vi "Param Sweep Dialog.vi"(8 "error in":errorcluster, 10 "Sweeps In":T1[](array[typedef])) -> (0 "error out":errorcluster, 1 "Cancelled?":bool, 2 "Sweeps out":T1[](array[typedef]), 4 "Movies to acquire":u32=1)   [LabVIEW 2023]
uses:
  Resources/Type Defs/Param Sweep.ctl
  896b73e1-52d9-41ed-b2a6-3a6588fcdd74.vi
panel:
  in  "Values":u32[](array[numeric])
  in  "Parameter":enum16{"Laser Power (mW)", "Exposure Time (ms)"}(ring)
  in  "Cancel":bool caption="Boolean 2"
  in  "Ok":bool caption="Boolean"
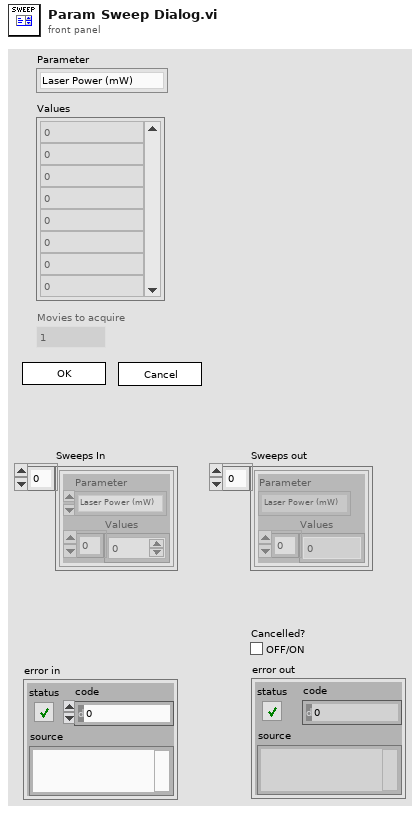
[diagram p1: front panel]
types:
  T1 = typedef "Param Sweep.ctl" = cluster{"Parameter":enum16{"Laser Power (mW)", "Exposure Time (ms)"}, "Values":u32[]}
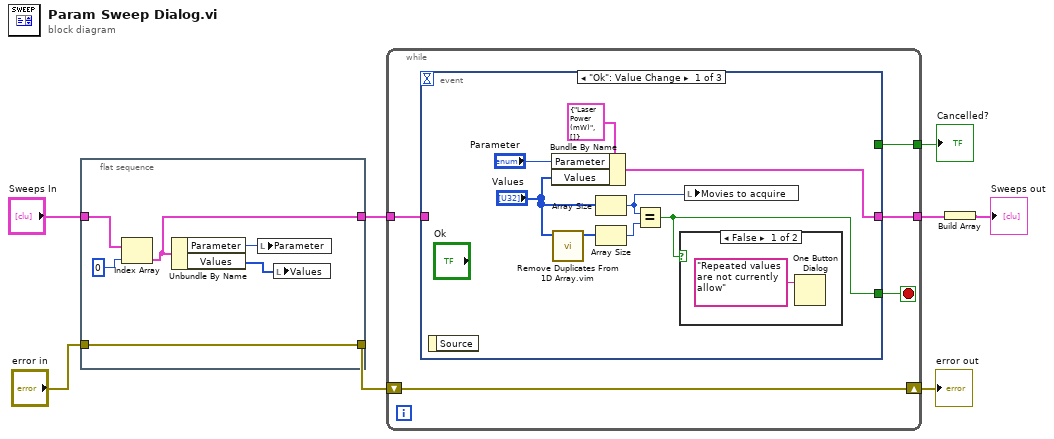
[diagram p0: block diagram]
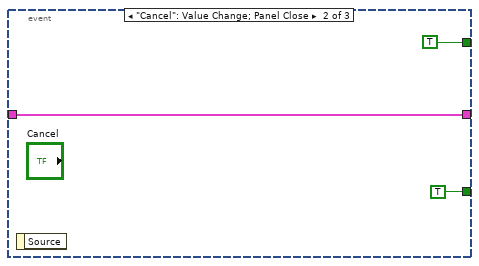
[diagram p3: hidden frame]
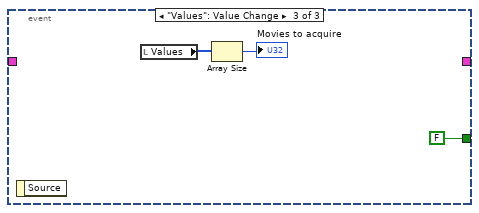
[diagram p4: hidden frame]
diagram:
  n1 = flat-sequence {
    tunnel: "Sweeps In" -> [w11]
    tunnel: "error in" -> [w12]
    tunnel: [w12] -> w6
    tunnel: [w9] -> w4
    frame #0 {
      n2 = Index Array(array=w11, index=0) -> (element=w9:T1)
      n3 = Unbundle By Name(w9) -> ("Parameter"=w14:enum16{"Laser Power (mW)", "Exposure Time (ms)"}, "Values"=w13:u32[])
      n4 = local write "Parameter"(w14) -> ()
      n5 = local write "Values"(w13) -> ()
    }
  }
  n6 = while {
    tunnel: [w18] -> w3
    shift-right: [w17] -> w8
    shift-left: w6 -> [w17]
    tunnel: [w16] -> w5
    tunnel: w4 -> [w15]
    stop <- w19 stop-if-true
    n7 = event shown="[0] \"Ok\": Value Change" {
      selector: _ -> [_ _ _]
      dyn-events: _ -> [_ _ _]
      timeout: _ -> [_ _ _]
      tunnel: [w21 TRUE FALSE] -> w19
      tunnel: [w25 w29 _] -> w18
      tunnel: [_ TRUE _] -> w16
      tunnel: w15 -> [_ w29 _]
      event "Ok": Value Change {
        n8 = event-data() -> ()  [unwired: 1 in, 1 out]
        n9 = Bundle By Name(cluster=T1 {"Parameter"=enum."Laser Power (mW)", "Values"=[]} ("Sweep"), "Parameter"="Parameter", "Values"="Values") -> (w25:T1)
        n10 = call "Remove Duplicates From 1D Array.vim"("array"="Values") -> ("array with duplicates removed"=w23:u32[])  [unwired: 10 in]
        n11 = Array Size(array="Values") -> (size(s)=w20:i32)
        n12 = Array Size(array=w23) -> (size(s)=w22:i32)
        n13 = Equal?(x=w20, y=w22) -> (x = y?=w21:bool)
        n14 = case shown="False" w21 {
          frame False {
            n15 = One Button Dialog(message="Repeated values are not currently allow") -> ()  [unwired: 1 in, 1 out]
          }
          frame True {
          }
        }
        n16 = local write "Movies to acquire"(w20) -> ()
      }
      event "Cancel": Value Change; Panel Close {
        n17 = event-data() -> ()  [unwired: 1 in, 1 out]
      }
      event "Values": Value Change {
        n18 = event-data() -> ()  [unwired: 1 in, 1 out]
        n19 = local read "Values"() -> (w33:u32[])
        n20 = Array Size(array=w33) -> (size(s)=→"Movies to acquire":i32)
      }
    }
  }
  "error out" <- w8
  "Cancelled?" <- w5
  n21 = Build Array(w3) -> (→"Sweeps out":T1[])
